vi "Test_Locate.vi"() -> ()   [LabVIEW 2019, in "Test_Maui.Config.lvclass"]
uses:
  Test_Maui.Config.lvclass
  lvsrc/Maui 1.0/Maui.Config/Maui.Config.lvclass
  <vilib>/addons/_JKI Toolkits/Caraya/classes/Assert/Assert.lvclass
  <vilib>/addons/_JKI Toolkits/Caraya/classes/Test/Test.lvclass
  <vilib>/addons/_JKI Toolkits/Caraya/classes/Assert/Assert Equal Value_Variant.vi
  <vilib>/addons/_JKI Toolkits/Caraya/classes/Assert/Assert False.vi
  <vilib>/addons/_JKI Toolkits/Caraya/classes/Assert/Assert True.vi
panel:
  in  "error in (no error)":errorcluster
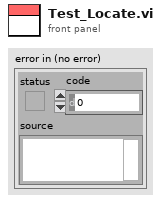
[diagram p1: front panel]
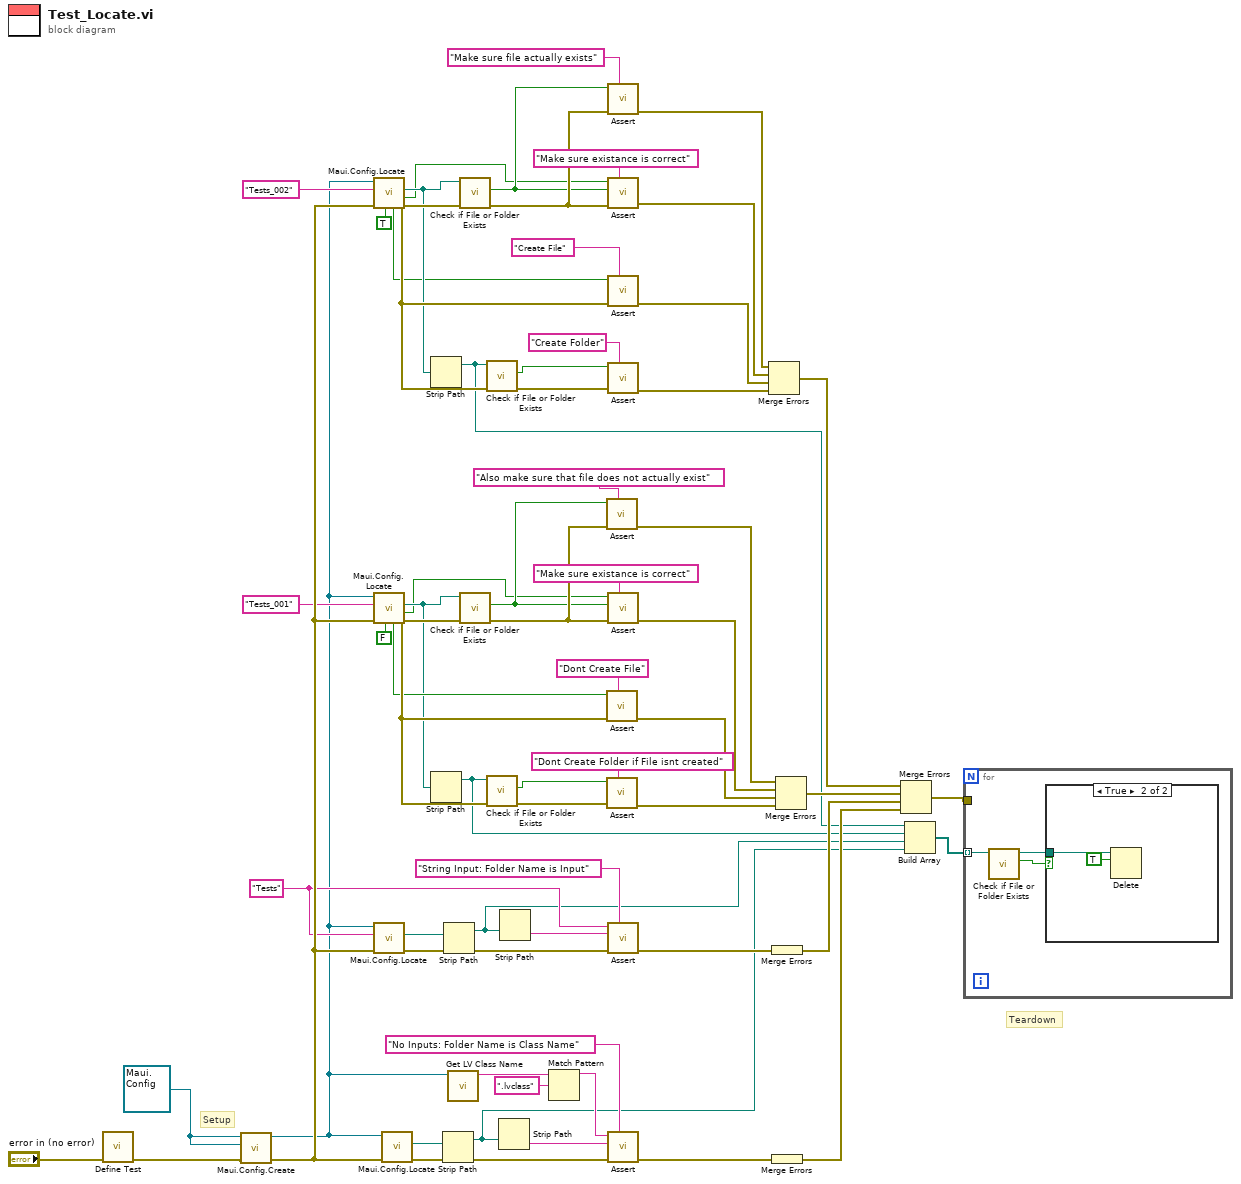
[diagram p0: block diagram]
diagram:
  w32 = "Tests" ("Application Name")
  w40 = refnum<class "Maui.Config.lvclass"> refnum ("Maui.Config in")
  # "Teardown"
  # "Setup"
  n1 = call <vilib>:"Define Test.vi"("error in (no error)"="error in (no error)") -> ("error out"=w64:errorcluster)  [unwired: 10 in]
  n2 = call "Maui.Config.Create.vi"("error in (no error)"=w64, "Owning Class"=w40, "Maui.Config in"=w40) -> ("error out"=w56:errorcluster, "Maui.Config out"=w9:refnum<class "Maui.Config.lvclass">)  [unwired: 7 in]
  n3 = call "Maui.Config.Locate.vi"("Create?"=TRUE, "error in (no error)"=w56, "Application Name"="Tests_002", "Maui.Config in"=w9) -> ("error out"=w57:errorcluster, "Exists?"=w13:bool, "Path"=w15:path, "Created?"=w14:bool)  [unwired: 3 in, 1 out]
  n4 = call "Maui.Config.Locate.vi"("Create?"=FALSE, "error in (no error)"=w56, "Application Name"="Tests_001", "Maui.Config in"=w9) -> ("error out"=w62:errorcluster, "Exists?"=w3:bool, "Path"=w24:path, "Created?"=w25:bool)  [unwired: 3 in, 1 out]
  n5 = call "Maui.Config.Locate.vi"("error in (no error)"=w56, "Application Name"=w32, "Maui.Config in"=w9) -> ("error out"=w63:errorcluster, "Path"=w34:path)  [unwired: 4 in, 3 out]
  n6 = call "Maui.Config.Locate.vi"("error in (no error)"=w56, "Maui.Config in"=w9) -> ("error out"=w65:errorcluster, "Path"=w39:path)  [unwired: 5 in, 3 out]
  n7 = Strip Path(path=w15) -> (stripped path=w7:path)  [unwired: 1 out]
  n8 = Strip Path(path=w24) -> (stripped path=w19:path)  [unwired: 1 out]
  n9 = Strip Path(path=w39) -> (stripped path=w5:path)  [unwired: 1 out]
  n10 = Strip Path(path=w34) -> (stripped path=w6:path)  [unwired: 1 out]
  n11 = call <vilib>:"Get LV Class Name.vi"("object"=w9) -> ("class name"=w35:string)  [unwired: 9 in, 1 out]
  n12 = call <vilib>:"Check if File or Folder Exists.vi"("error in (no error)"=w57, "path"=w15) -> ("error out"=w59:errorcluster, "file or folder exists?"=w18:bool)  [unwired: 7 in, 1 out]
  n13 = call <vilib>:"Check if File or Folder Exists.vi"("error in (no error)"=w62, "path"=w24) -> ("error out"=w60:errorcluster, "file or folder exists?"=w21:bool)  [unwired: 7 in, 1 out]
  n14 = call <vilib>:"Check if File or Folder Exists.vi"("error in (no error)"=w57, "path"=w7) -> ("error out"=w58:errorcluster, "file or folder exists?"=w16:bool)  [unwired: 7 in, 1 out]
  n15 = call <vilib>:"Check if File or Folder Exists.vi"("error in (no error)"=w62, "path"=w19) -> ("error out"=w61:errorcluster, "file or folder exists?"=w23:bool)  [unwired: 7 in, 1 out]
  n16 = Strip Path(path=w5) -> (name=w38:string)  [unwired: 1 out]
  n17 = Strip Path(path=w6) -> (name=w33:string)  [unwired: 1 out]
  n18 = Match Pattern(string=w35, regular expression=".lvclass") -> (before substring=w36:string)  [unwired: 1 in, 3 out]
  n19 = call-poly <vilib>:"Assert.vi"("Label"="Also make sure that file does not actually exist", "error in (no error)"=w60, "False?"=w21) -> ("error out"=w51:errorcluster)  [unwired: 8 in]
  n20 = call-poly <vilib>:"Assert.vi"("Label"="Dont Create File", "error in (no error)"=w62, "False?"=w25) -> ("error out"=w49:errorcluster)  [unwired: 8 in]
  n21 = call-poly <vilib>:"Assert.vi"("Label"="Dont Create Folder if File isnt created", "error in (no error)"=w61, "False?"=w23) -> ("error out"=w48:errorcluster)  [unwired: 8 in]
  n22 = call-poly <vilib>:"Assert.vi"("Label"="Make sure file actually exists", "error in (no error)"=w59, "True?"=w18) -> ("error out"=w52:errorcluster)  [unwired: 8 in]
  n23 = call-poly <vilib>:"Assert.vi"("Label"="Make sure existance is correct", "error in (no error)"=w59, "Y"=w18, "X"=w13) -> ("error out"=w53:errorcluster)  [unwired: 7 in]
  n24 = call-poly <vilib>:"Assert.vi"("Label"="Create File", "error in (no error)"=w57, "True?"=w14) -> ("error out"=w54:errorcluster)  [unwired: 8 in]
  n25 = call-poly <vilib>:"Assert.vi"("Label"="Create Folder", "error in (no error)"=w58, "True?"=w16) -> ("error out"=w55:errorcluster)  [unwired: 8 in]
  n26 = call-poly <vilib>:"Assert.vi"("Label"="Make sure existance is correct", "error in (no error)"=w60, "Y"=w21, "X"=w3) -> ("error out"=w50:errorcluster)  [unwired: 7 in]
  n27 = call-poly <vilib>:"Assert.vi"("Label"="String Input: Folder Name is Input", "error in (no error)"=w63, "Y"=w33, "X"=w32) -> ("error out"=w47:errorcluster)  [unwired: 7 in]
  n28 = call-poly <vilib>:"Assert.vi"("Label"="No Inputs: Folder Name is Class Name" ("Label (VI Title)"), "error in (no error)"=w65, "Y"=w38, "X"=w36) -> ("error out"=w46:errorcluster)  [unwired: 7 in]
  n29 = Merge Errors(w52, w53, w54, w55) -> (w45:errorcluster)
  n30 = Merge Errors(w47) -> (w43:errorcluster)
  n31 = Merge Errors(w46) -> (w42:errorcluster)
  n32 = Merge Errors(w51, w50, w49, w48) -> (w44:errorcluster)
  n33 = Merge Errors(w45, w44, w43, w42) -> (w4:errorcluster)
  n34 = Build Array(w7, w19, w6, w5) -> (w30:path[])
  n35 = for {
    tunnel: w30 -> [w68] mode=indexing
    tunnel: w4 -> [_]
    n36 = call <vilib>:"Check if File or Folder Exists.vi"("path"=w68) -> ("file or folder exists?"=w67:bool, "dup path"=w66:path)  [unwired: 8 in, 1 out]
    n37 = case shown="True" w67 {
      tunnel: w66 -> [_ w70]
      frame False {
      }
      frame True {
        n38 = Delete(path (use dialog)=w70, entire hierarchy (F)=TRUE) -> ()  [unwired: 3 in, 3 out]
      }
    }
  }
